vi "Get ROI from Display.vi"(7 "Display Index":i32) -> (8 "Image Out":u16[][](array[numeric]))   [LabVIEW 2016]
uses:
  Display Module Custom Controls/ROI Descriptor.ctl
  <vilib>/vision/Image Controls.llb/IMAQ Image.ctl
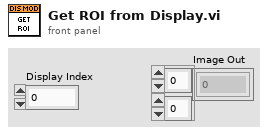
[diagram p1: front panel]
types:
  T1 = typedef "IMAQ Image.ctl" = refnum<image>
  T2 = typedef "ROI Descriptor.ctl" = cluster{"Global Rectangle":i32[], "Contours":cluster{"Contour Type":u32, "ROI Type":u32, "Points":i32[]}[]}
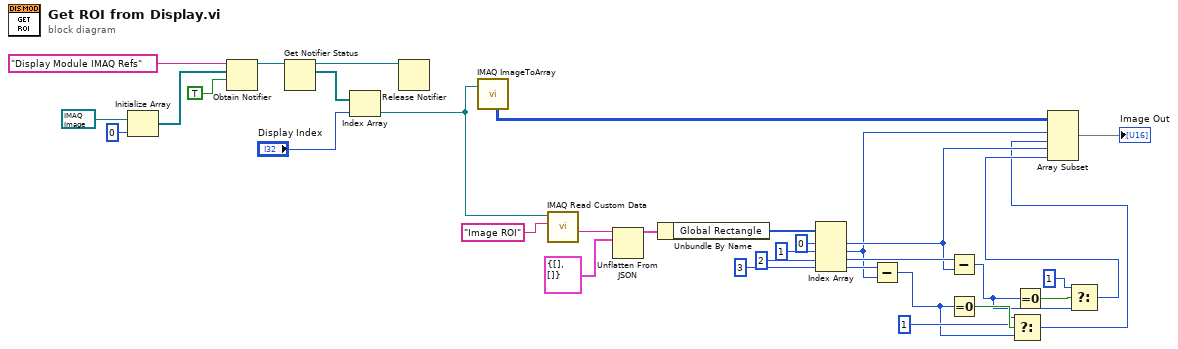
[diagram p0: block diagram]
diagram:
  n1 = Initialize Array(T1 refnum ("New Image"), 0 ("dimension size")) -> (w6:T1[])
  n2 = Obtain Notifier(name (unnamed)="Display Module IMAQ Refs", notification data type=w6, create if not found? (T)=TRUE) -> (notifier out=w5:refnum<notifier>)  [unwired: 1 in, 2 out]
  n3 = Get Notifier Status(notifier=w5) -> (notifier out=w1:refnum<notifier>, current notification=w4:T1[])  [unwired: 1 in, 3 out]
  n4 = Index Array(array=w4, index="Display Index") -> (element=w3:T1)
  n5 = Release Notifier(notifier=w1) -> ()  [unwired: 2 in, 3 out]
  n6 = call "IMAQ ImageToArray"("Image"=w3) -> ("Image Pixels (U16)"=w24:u16[][])  [unwired: 3 in, 4 out]
  n7 = call "IMAQ Read Custom Data"("Key"="Image ROI", "Image"=w3) -> ("Custom Data Out"=w32:string)  [unwired: 7 in, 2 out]
  n8 = Unflatten From JSON(JSON string=w32, type and defaults=T2 {"Global Rectangle"=[], "Contours"=[]} ("Image ROI Descriptor")) -> (value=w30:T2)  [unwired: 5 in, 1 out]
  n9 = Unbundle By Name(w30) -> ("Global Rectangle"=w29:i32[])
  n10 = Index Array(array=w29, index #1=0 ("index"), index #2=1 ("index"), index #3=2 ("index"), index #4=3 ("index")) -> (element #1=w21:i32, element #2=w20:i32, element #3=w23:i32, element #4=w22:i32)
  n11 = Subtract(x=w22, y=w20) -> (x-y=w15:i32)
  n12 = Subtract(x=w23, y=w21) -> (x-y=w14:i32)
  n13 = Equal To 0?(x=w15) -> (x = 0?=w19:bool)
  n14 = Select(t=1 ("index"), s=w19, f=w15) -> (s? t:f=w12:i32)
  n15 = Equal To 0?(x=w14) -> (x = 0?=w18:bool)
  n16 = Select(t=1 ("index"), s=w18, f=w14) -> (s? t:f=w13:i32)
  n17 = Array Subset(array=w24, index (row)=w20, length (row)=w12, index (col)=w21, length (col)=w13) -> (→"Image Out":u16[][])
